vi "Bandpass Filter Cont.vi"(0 "DataFilter in":refnum<class "DataFilter.lvclass">, 1 "X":dbl[](array[numeric]), 2 "low cutoff freq: fl":dbl=0.12500000000000006 format="%0.4f", 3 "high cutoff freq: fh":dbl=0.45000000000000007 format="%0.2f", 4 "sampling freq: fs":dbl=1.0 format="%0.2f", 5 "error in (no error)":errorcluster, 7 "init/cont (init:F)":bool=TRUE, 9 "Overlap Length":dbl=200.0) -> (14 "DataFilter out":refnum<class "DataFilter.lvclass">, 15 "Filtered X":dbl[](array[numeric]), 19 "error out":errorcluster)   [LabVIEW 2010, in "DataFilter.lvclass"]
uses:
  DataFilter.lvclass
  <vilib>/Analysis/3filter.llb/Filter Passband Type.ctl
  <vilib>/Analysis/3filter.llb/Butterworth Filter (DBL).vi
  <vilib>/Analysis/NI_AALBase.lvlib
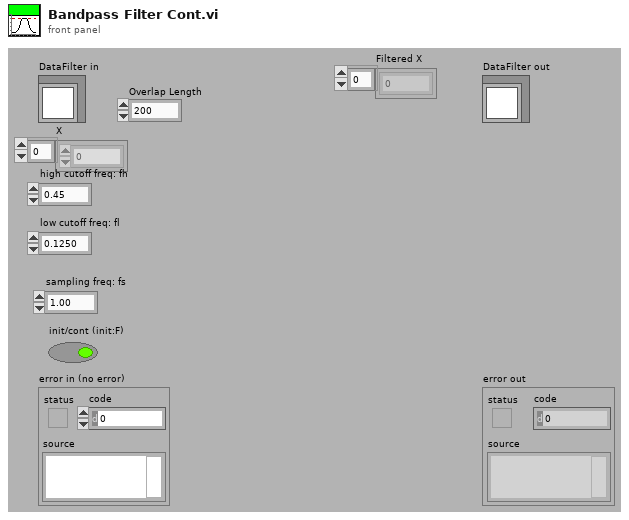
[diagram p1: front panel]
types:
  T1 = typedef "NI_AALBase.lvlib/Filter Passband Type.ctl" = enum32{"Lowpass", "Highpass", "Bandpass", "Bandstop"}
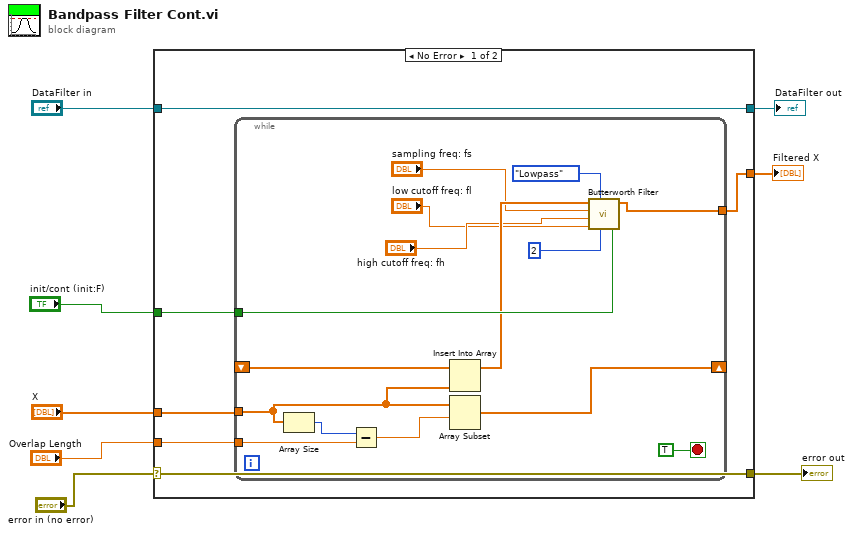
[diagram p0: block diagram]
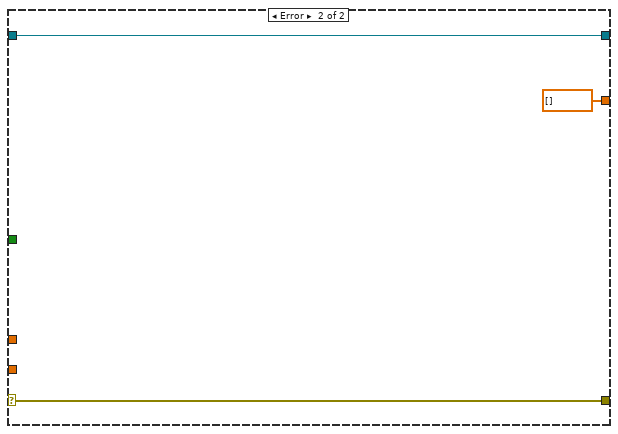
[diagram p2: hidden frame]
diagram:
  n1 = case shown="No Error" "error in (no error)" {
    selector: "error in (no error)" -> [w14 w32]
    tunnel: [w14 w32] -> w7
    tunnel: [w12 w31] -> w5
    tunnel: "DataFilter in" -> [w12 w31]
    tunnel: "X" -> [w13 _]
    tunnel: "init/cont (init:F)" -> [w11 _]
    tunnel: [w10 dbl[] [] ("Filtered X")] -> w2
    tunnel: "Overlap Length" -> [w9 _]
    frame No Error {
      n2 = while {
        tunnel: w13 -> [w20]
        tunnel: w11 -> [w27]
        tunnel: [w26] -> w10
        tunnel: w9 -> [w23]
        shift-right: [w22] -> _
        shift-left: _ -> [w19]
        stop <- TRUE stop-if-true
        n3 = Array Size(array=w20) -> (size(s)=w25:i32)
        n4 = Subtract(x=w25, y=w23) -> (x-y=w24:dbl)
        n5 = Insert Into Array(array=w19, new element=w20) -> (w21:dbl[])  [unwired: 1 in]
        n6 = Array Subset(array=w20, index=w24) -> (w22:dbl[])  [unwired: 1 in]
        n7 = call-poly <vilib>:"Butterworth Filter.vi"("init/cont (init:F)"=w27, "order"=2, "filter type"=Filter_Passband_Type."Lowpass", "low cutoff freq: fl"="low cutoff freq: fl", "high cutoff freq: fh"="high cutoff freq: fh", "sampling freq: fs"="sampling freq: fs", "X"=w21) -> ("Filtered X"=w26:dbl[])  [unwired: 1 in, 1 out]
      }
    }
    frame Error {
    }
  }
  "error out" <- w7
  "DataFilter out" <- w5
  "Filtered X" <- w2
